vi "remove pubsub mappings by module.vi"(10 "module id":string, 11 "streams in":T1) -> (3 "streams out":T1)   [LabVIEW 2013, in "engine configuration.lvclass"]
uses:
  engine configuration.lvclass
  simple mapping.ctl
  module channel pairings.ctl
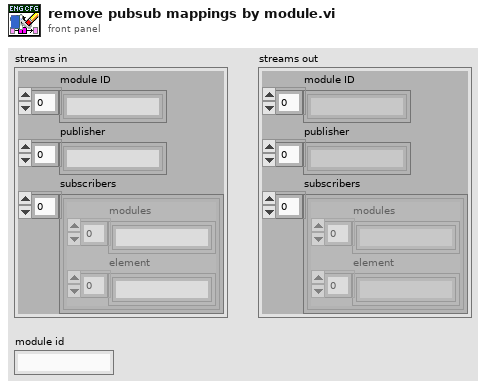
[diagram p1: front panel]
types:
  T1 = typedef "engine configuration.lvclass/simple mapping.ctl" = cluster{"module ID":string[], "publisher":string[], "subscribers":T2[]}
  T2 = typedef "engine configuration.lvclass/module channel pairings.ctl" = cluster{"modules":string[], "element":string[]}
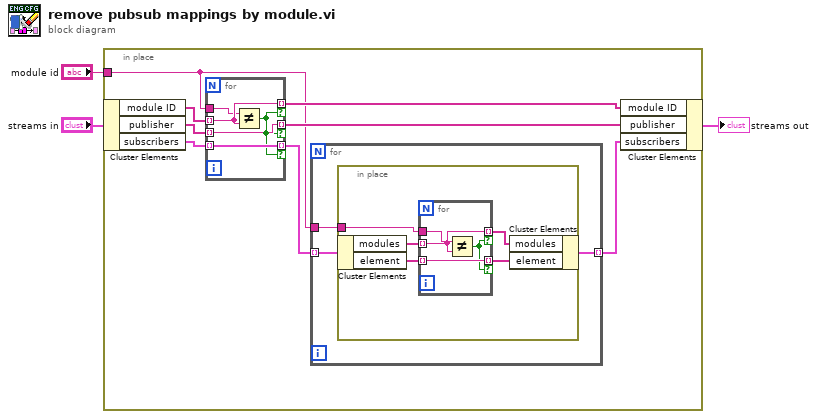
[diagram p0: block diagram]
diagram:
  n1 = in-place {
    in-place-border: "module id" -> [w7]
    n2 = in-place-cluster #1("streams in") -> ("module ID"=w11:string[], "publisher"=w10:string[], "subscribers"=w6:T2[])
    n3 = for {
      tunnel: w11 -> [w27] mode=indexing
      tunnel: w10 -> [w28] mode=indexing
      tunnel: [w27] -> w9 mode=indexing if=w24
      tunnel: [w28] -> w8 mode=indexing if=w24
      tunnel: w7 -> [w26]
      tunnel: [w25] -> w5 mode=indexing if=w24
      tunnel: w6 -> [w25] mode=indexing
      n4 = Not Equal?(x=w26, y=w27) -> (x != y?=w24:bool)
    }
    n5 = for {
      tunnel: w7 -> [w12]
      tunnel: w5 -> [w14] mode=indexing
      tunnel: [w13] -> w4 mode=indexing
      n6 = in-place {
        in-place-border: w12 -> [w19]
        n7 = in-place-cluster #2(w14) -> ("modules"=w18:string[], "element"=w16:string[])
        n8 = for {
          tunnel: w19 -> [w23]
          tunnel: w18 -> [w22] mode=indexing
          tunnel: [w22] -> w17 mode=indexing if=w20
          tunnel: w16 -> [w21] mode=indexing
          tunnel: [w21] -> w15 mode=indexing if=w20
          n9 = Not Equal?(x=w23, y=w22) -> (x != y?=w20:bool)
        }
        n10 = in-place-cluster #2("modules"=w17, "element"=w15) -> (w13:T2)
      }
    }
    n11 = in-place-cluster #1("module ID"=w9, "publisher"=w8, "subscribers"=w4) -> (→"streams out":T1)
  }
